vi "Image Averaging.vi"() -> ()   [LabVIEW 2014]
doc: "This example shows how to use image averaging to improve the signal/noise ratio of noisy images."
uses:
  <vilib>/vision/NI_Vision_Development_Module.lvlib
panel:
  out "Src":T1(plugin-control)
  out "Accumulated":i32
  out "Averaged":T1(plugin-control)
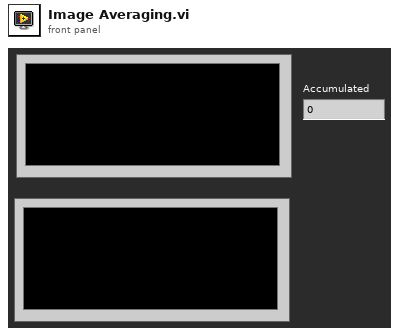
[diagram p1: front panel]
types:
  T1 = typedef "IMAQ Image.ctl" = refnum<image>
  T2 = typedef "Image Type" = u32
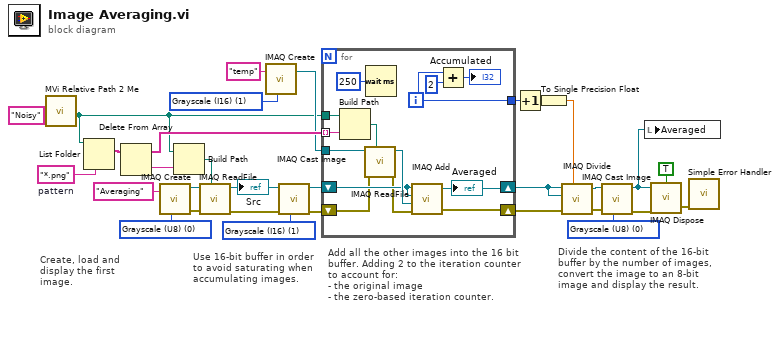
[diagram p0: block diagram]
diagram:
  w1 = "*.png"  # pattern
  w12 = T2 1 items=["Grayscale (U8)", "Grayscale (I16)", "Grayscale (SGL)", "Complex (CSG)", "RGB (U32)", "HSL (U32)", "RGB (U64)", "Grayscale (U16)"] ("Image Type")
  w13 = T2 0 items=["Grayscale (U8)", "Grayscale (I16)", "Grayscale (SGL)", "Complex (CSG)", "RGB (U32)", "HSL (U32)", "RGB (U64)", "Grayscale (U16)"] ("Image Type")
  w22 = T2 1 items=["Grayscale (U8)", "Grayscale (I16)", "Grayscale (SGL)", "Complex (CSG)", "RGB (U32)", "HSL (U32)", "RGB (U64)", "Grayscale (U16)"] ("Image Type")
  w24 = T2 0 items=["Grayscale (U8)", "Grayscale (I16)", "Grayscale (SGL)", "Complex (CSG)", "RGB (U32)", "HSL (U32)", "RGB (U64)", "Grayscale (U16)"] ("Image Type")
  # "Add all the other images into the 16 bit buffer. Adding 2 to the iteration counter to account for: \n- the original image\n- the zero-based iteration counter."
  # "Use 16-bit buffer in order to avoid saturating when accumulating images."
  # "Divide the content of the 16-bit buffer by the number of images, convert the image to an 8-bit image and display the result."
  # "Create, load and display the first image."
  n1 = call "MVi Relative Path 2 Me.vi"("Relative Path"="Noisy" ("name or relative path")) -> ("Appended Dir"=w5:path)  [unwired: 5 in, 1 out]
  n2 = List Folder(path=w5, pattern=w1) -> (filenames=w18:string[])  [unwired: 2 in, 3 out]
  n3 = Delete From Array(array=w18) -> (deleted portion=w19:string, array with subset deleted=w31:string[])  [unwired: 2 in]
  n4 = call "IMAQ Create"("Image Name"="Averaging", "Image Type"=w24) -> ("New Image"=w26:T1, "error out"=w20:errorcluster)  [unwired: 3 in]
  n5 = Build Path(base path=w5, name or relative path=w19) -> (appended path=w25:path)
  n6 = call "IMAQ ReadFile"("File Path"=w25, "error in (no error)"=w20, "Image"=w26) -> ("error out"=w28:errorcluster, "Image Out"=w4:T1)  [unwired: 4 in, 3 out]
  "Src" <- w4
  n7 = call "IMAQ Create"("Image Name"="temp", "Image Type"=w22) -> ("New Image"=w30:T1)  [unwired: 3 in, 1 out]
  n8 = call "IMAQ Cast Image"("Image Type"=w12, "error in (no error)"=w28, "Image Src"=w4) -> ("error out"=w9:errorcluster, "Image Dst Out"=w11:T1)  [unwired: 7 in]
  n9 = for {
    tunnel: w5 -> [w45]
    tunnel: w31 -> [w44] mode=indexing
    tunnel: w30 -> [w42]
    shift-right: [w39] -> w16
    shift-left: w11 -> [w40]
    tunnel: [w35] -> w15
    shift-right: [w38] -> w8
    shift-left: w9 -> [w37]
    i -> [w35]
    n10 = Build Path(base path=w45, name or relative path=w44) -> (appended path=w43:path)
    n11 = call "IMAQ ReadFile"("File Path"=w43, "error in (no error)"=w37, "Image"=w42) -> ("error out"=w36:errorcluster, "Image Out"=w41:T1)  [unwired: 4 in, 3 out]
    n12 = Wait (ms)(milliseconds to wait=u32 250) -> ()  [unwired: 1 out]
    n13 = call "IMAQ Add"("Image Src A"=w40, "Image Dst"=w40, "Image Src B"=w41, "error in (no error)"=w36) -> ("Image Dst Out"=w39:T1, "error out"=w38:errorcluster)  [unwired: 3 in]
    "Averaged" <- w39
    n14 = Add(x=w35, y=2) -> (x+y=→"Accumulated":i32)
  }
  n15 = Increment(x=w15) -> (x+1=w14:i32)
  n16 = To Single Precision Float(number=w14) -> (single precision float=w10:sgl)
  n17 = call "IMAQ Divide"("Image Src A"=w16, "Constant"=w10, "Image Dst"=w16, "error in (no error)"=w8) -> ("Image Dst Out"=w17:T1, "error out"=w7:errorcluster)  [unwired: 3 in]
  n18 = call "IMAQ Cast Image"("Image Type"=w13, "error in (no error)"=w7, "Image Src"=w17) -> ("error out"=w27:errorcluster, "Image Dst Out"=w29:T1)  [unwired: 7 in]
  n19 = local write "Averaged"(w29) -> ()
  n20 = call "IMAQ Dispose"("All Images? (No)"=TRUE, "Image"=w29, "error in (no error)"=w27) -> ("error out"=w3:errorcluster)  [unwired: 3 in]
  n21 = call <vilib>:"Simple Error Handler.vi"("error in (no error)"=w3) -> ()  [unwired: 4 in, 5 out]
